vi "v5.1.vi"() -> ()   [LabVIEW 2018]
uses:
  <vilib>/DAQmx/read.llb/DAQmx Read (Analog 1D DBL NChan 1Samp).vi
  <extravilib>/ChannelInstances/High Speed Stream-c(a[.](c(dbl,dbl,dbl,dbl)),stamp,a[.](dbl),c(dbl,dbl,dbl,dbl,dbl,dbl,dbl))/_Read For Replicate.vi
  <extravilib>/ChannelInstances/High Speed Stream-c(a[.](c(dbl,dbl,dbl,dbl)),stamp,a[.](dbl),c(dbl,dbl,dbl,dbl,dbl,dbl,dbl))/Instantiate.vi
  <extravilib>/ChannelInstances/High Speed Stream-c(a[.](c(dbl,dbl,dbl,dbl)),stamp,a[.](dbl),c(dbl,dbl,dbl,dbl,dbl,dbl,dbl))/)Channel.vi
  <extravilib>/ChannelInstances/High Speed Stream-c(a[.](c(dbl,dbl,dbl,dbl)),stamp,a[.](dbl),c(dbl,dbl,dbl,dbl,dbl,dbl,dbl))/Abort Signal/Init Signal.vi
  <vilib>/Utility/file.llb/Write Delimited Spreadsheet (string).vi
  <vilib>/DAQmx/create/channels.llb/DAQmx Create Channel (AI-Temperature-Thermocouple).vi
  <vilib>/DAQmx/configure/timing.llb/DAQmx Timing (Sample Clock).vi
  <vilib>/DAQmx/miscellaneous.llb/DAQmx Fill In Error Info.vi
  <extravilib>/ChannelInstances/High Speed Stream-c(a[.](c(dbl,dbl,dbl,dbl)),stamp,a[.](dbl),c(dbl,dbl,dbl,dbl,dbl,dbl,dbl)).lvlib
  <resource>/objmgr/daqmx.rc
panel:
  in  "stop":bool
  in  "Species List":string[][](table)=[["Custom", "9999999999"], ["Methanol", "6.47"], ["Butanol", "11.2"], ["Diesel", "14.5"], ["Gasoline", "14.7"], ["Propane", "15.67"], ["Methane", "13.19"], ["Hydrogen", "34.3"], ["Ammonia", "6.0466"], ["Pentane", "15.32"], ["Butane", "14.98"], ["Hexane", "15.24"], ["Ethanol", "9"]]
  in  "Tab Control":enum32{"Live Data", "AFR Info", "Setup Lines"}(tab)
  out "Flowrate Data":T1(array[cluster])
  out "AFR Display":T2(array[cluster])
  in  "Line Setup":T3(array[cluster])
  out "Actual Sample Rate":dbl
  out "Export Timestamp":timestamp format="%<%H:%M:%S>T"
  out "Rig Temperatures":T4
  out "UI Timestamp":timestamp format="%<%X\n%x>T"
  out "DAQ Timestamp":timestamp format="%<%H:%M:%S>T"
  in  "file path (dialog if empty)":path
  out "Export Loop Status":T5(ring)
  in  "Start Recording?":bool
  in  "Stop Recording?":bool
  in  "Flowrate Control":dbl
  out "Aquisition Loop Status":T6(ring)
  in  "OK Button":bool
  in  "DAQ Properties":cluster{"Sample Rate [Hz]":dbl}={"Sample Rate [Hz]"=1.0} {"Sample Rate [Hz]" min=0.1 max=10000.0 step=0.1}
  # "Live \n Live Line Data"
  # "Air-to-Fuel Ratios for each Line"
  # "Line Setup"
  # "Rig Temperatures [ °C]"
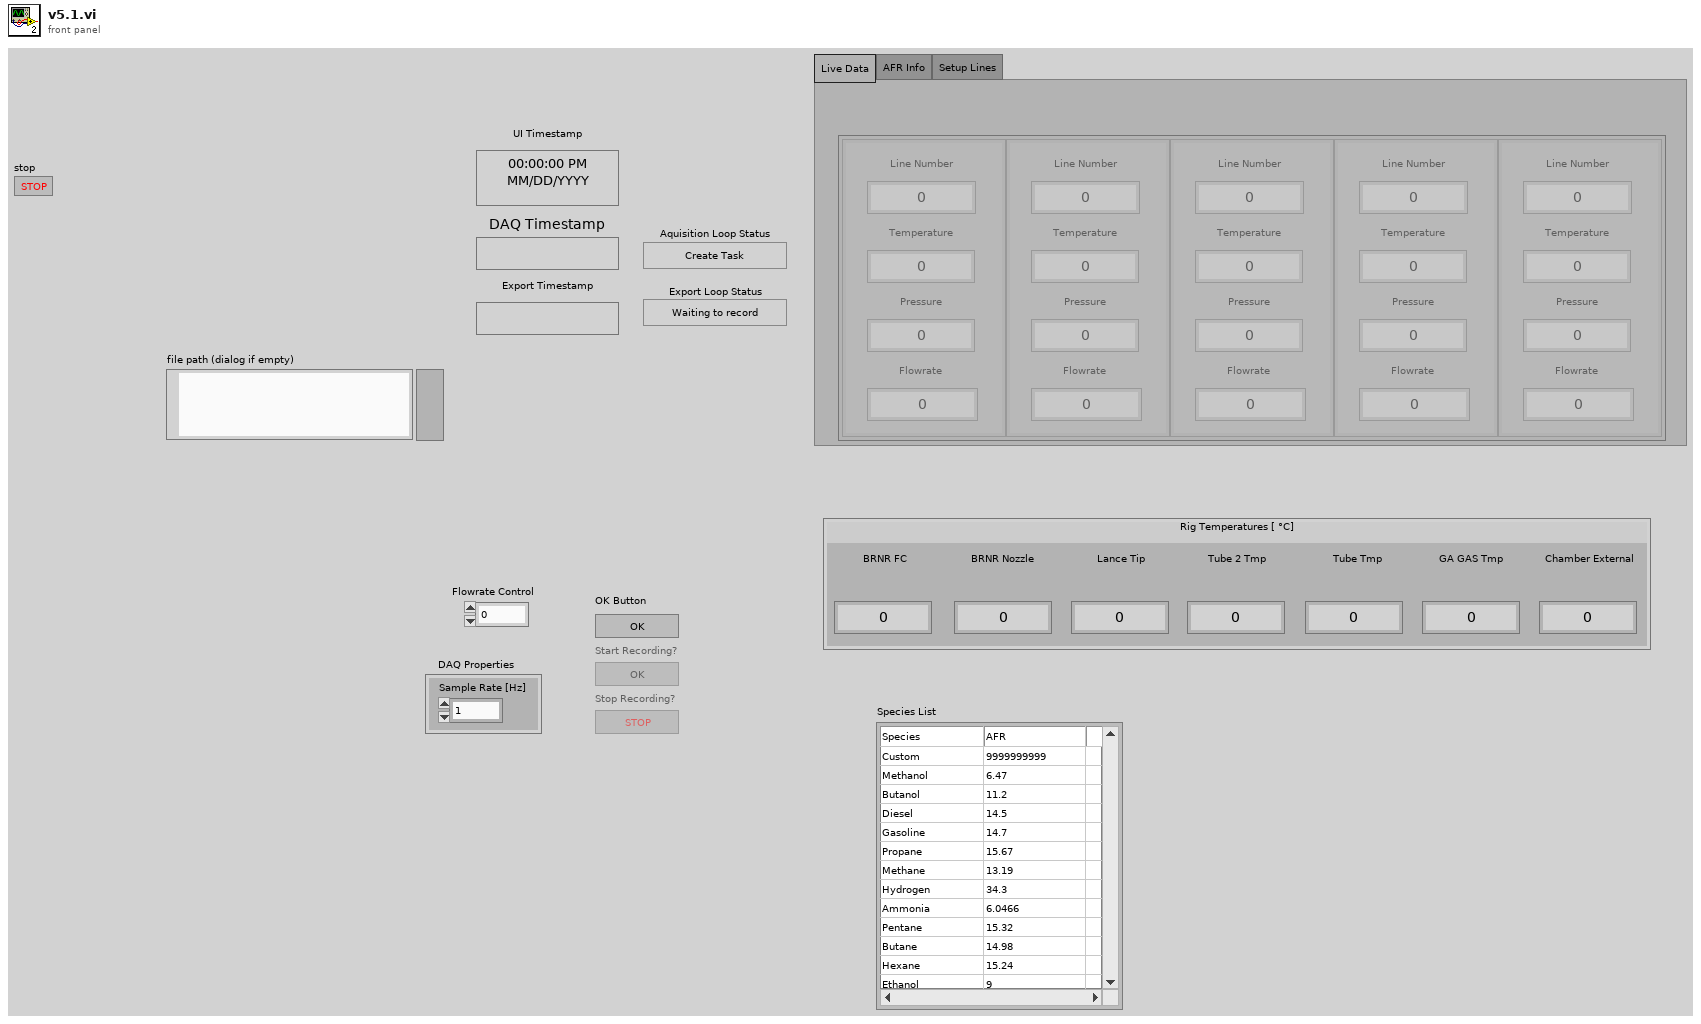
[diagram p1: front panel]
types:
  T1 = cluster{"Line Number":dbl, "Temperature":dbl, "Pressure":dbl, "Flowrate":dbl}[]
  T2 = cluster{"Line Number":i32, "AFR":dbl, "Species":enum16{"Methanol", "Ethanol", "Butanol", "Diesel", "Gasoline", "Propane", "Methane", "Hydrogen", "Pentane", "Butane", "Hexane", "Custom"}}[]
  T3 = cluster{"Custom AFR":dbl, "Species":enum16{"Methanol", "Ethanol", "Butanol", "Diesel", "Gasoline", "Propane", "Methane", "Hydrogen", "Pentane", "Butane", "Hexane", "Custom"}}[]
  T4 = cluster{"BRNR FC":dbl, "BRNR Nozzle":dbl, "Lance Tip":dbl, "Tube 2 Tmp":dbl, "Tube Tmp":dbl, "GA GAS Tmp":dbl, "Chamber External":dbl}
  T5 = enum16{"Waiting to record", "Creating Spreadsheet", "Recording", "Finished Recording"}
  T6 = enum16{"Create Task", "Change Settings", "Check Settings", "Read Data", "End Task"}
  T7 = enum8{"Enabled", "Disabled", "Disabled and Grayed Out"}
  T8 = cluster{"Line":i32, "AFR":dbl, "Species":enum16{"Methanol", "Ethanol", "Butanol", "Diesel", "Gasoline", "Propane", "Methane", "Hydrogen", "Pentane", "Butane", "Hexane", "Custom"}}
  T9 = enum16{"Methanol", "Ethanol", "Butanol", "Diesel", "Gasoline", "Propane", "Methane", "Hydrogen", "Pentane", "Butane", "Hexane", "Custom"}
  T10 = cluster{"Flowrate Data":cluster{"Line Number":dbl, "Temperature":dbl, "Pressure":dbl, "Flowrate":dbl}[], "Current Time":timestamp, "DAQmx Data":dbl[], "Rig Temperatures":cluster{"BRNR FC":dbl, "BRNR Nozzle":dbl, "Lance Tip":dbl, "Tube 2 Tmp":dbl, "Tube Tmp":dbl, "GA GAS Tmp":dbl, "Chamber External Temp":dbl}}
  T11 = cluster{"BRNR FC":dbl, "BRNR Nozzle":dbl, "Lance Tip":dbl, "Tube 2 Tmp":dbl, "Tube Tmp":dbl, "GA GAS Tmp":dbl, "Chamber External Temp":dbl}
  T12 = typedef "High Speed Stream-c(a[.](c(dbl,dbl,dbl,dbl)),stamp,a[.](dbl),c(dbl,dbl,dbl,dbl,dbl,dbl,dbl)).lvlib/)Channel.ctl" = refnum<queue>
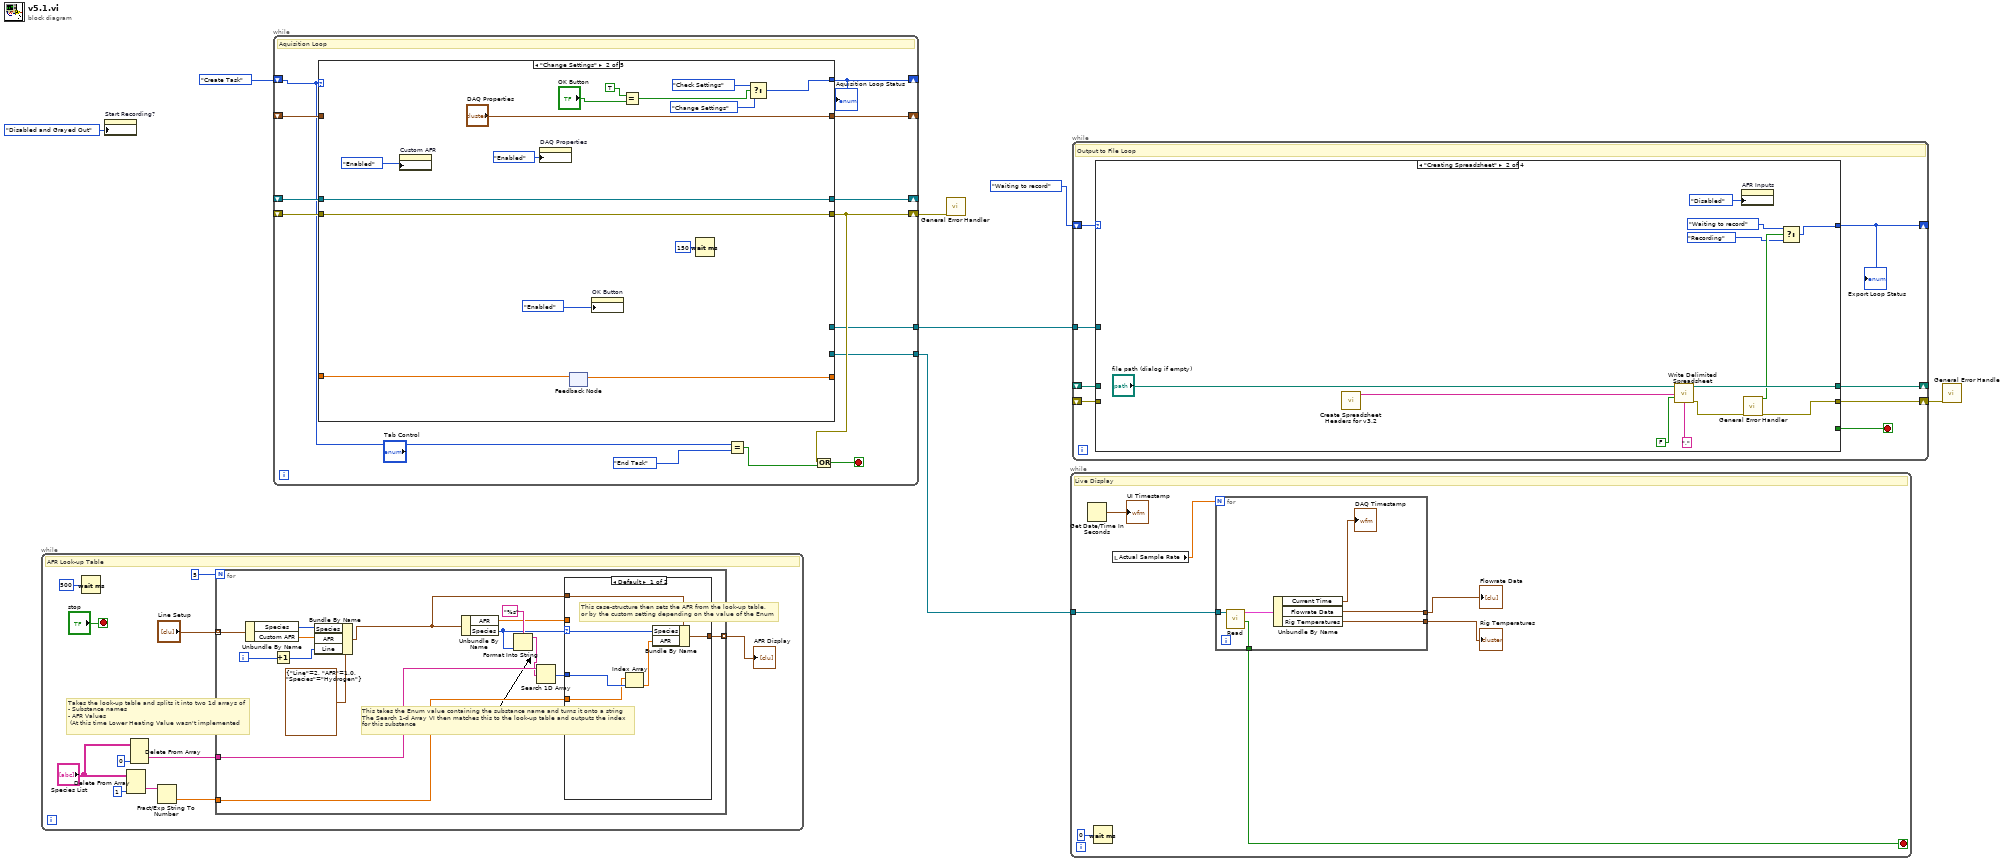
[diagram p0: block diagram]
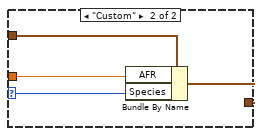
[diagram p2: hidden frame]
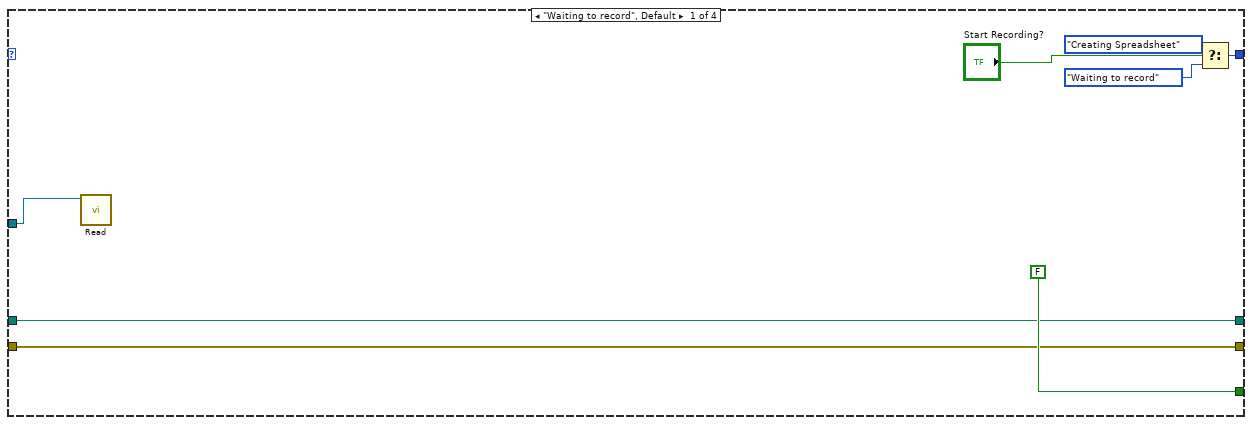
[diagram p3: hidden frame]
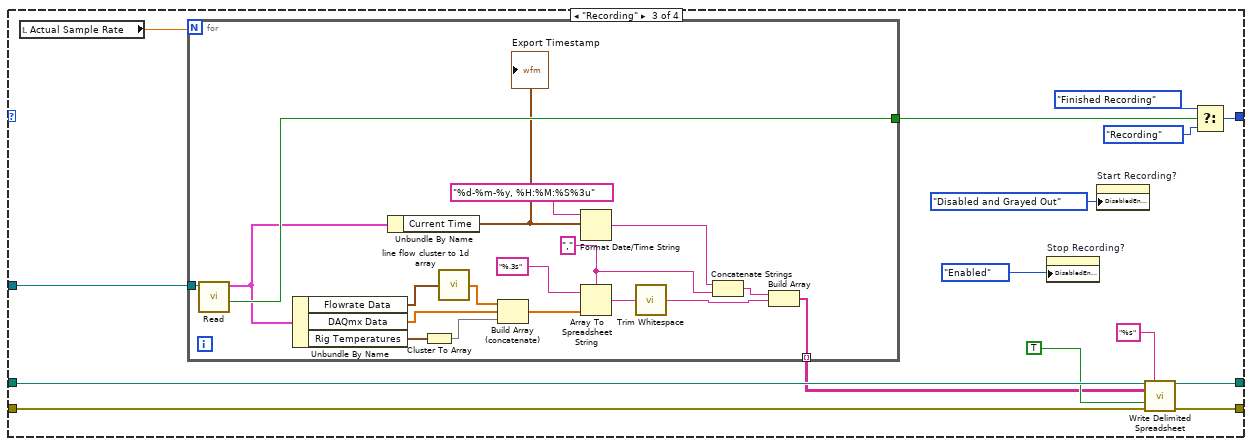
[diagram p4: hidden frame]
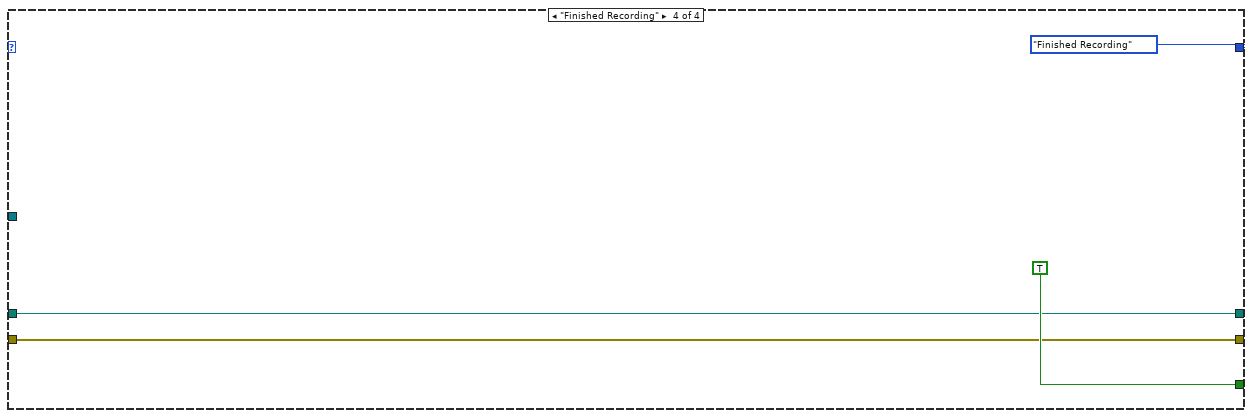
[diagram p5: hidden frame]
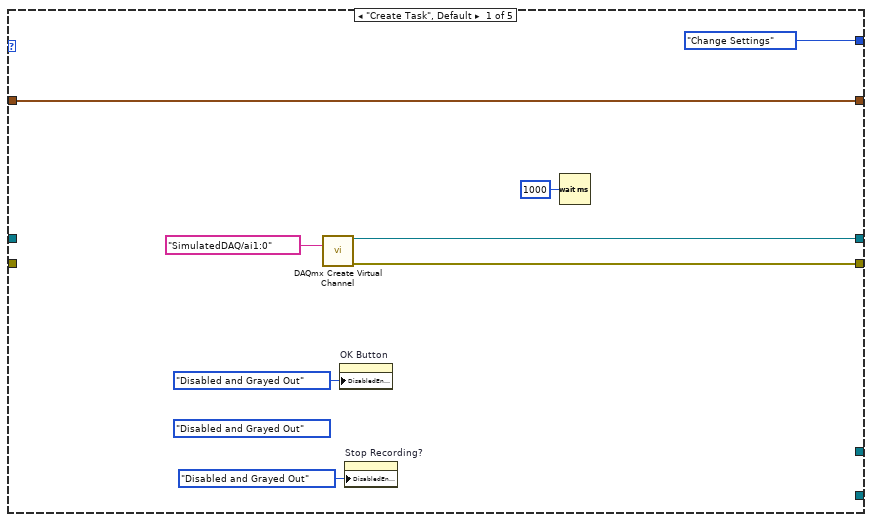
[diagram p6: hidden frame]
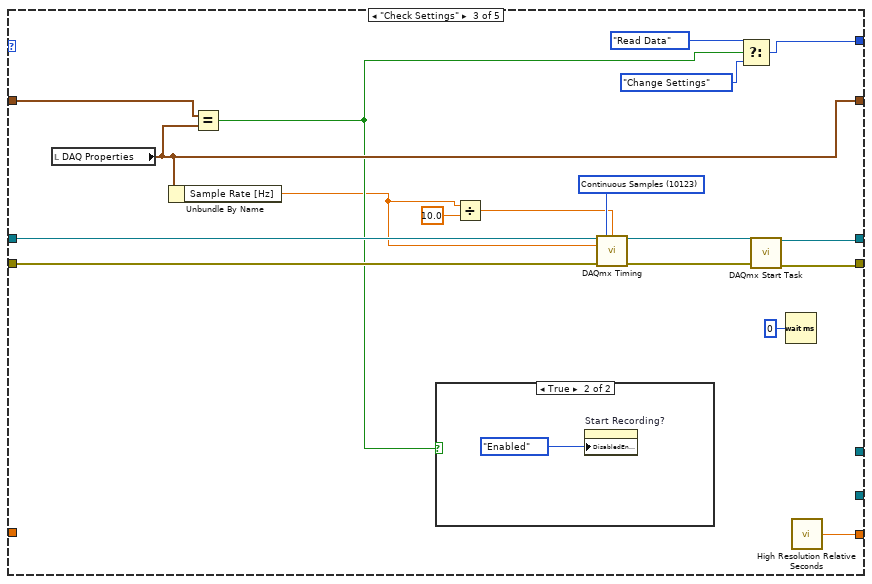
[diagram p7: hidden frame]
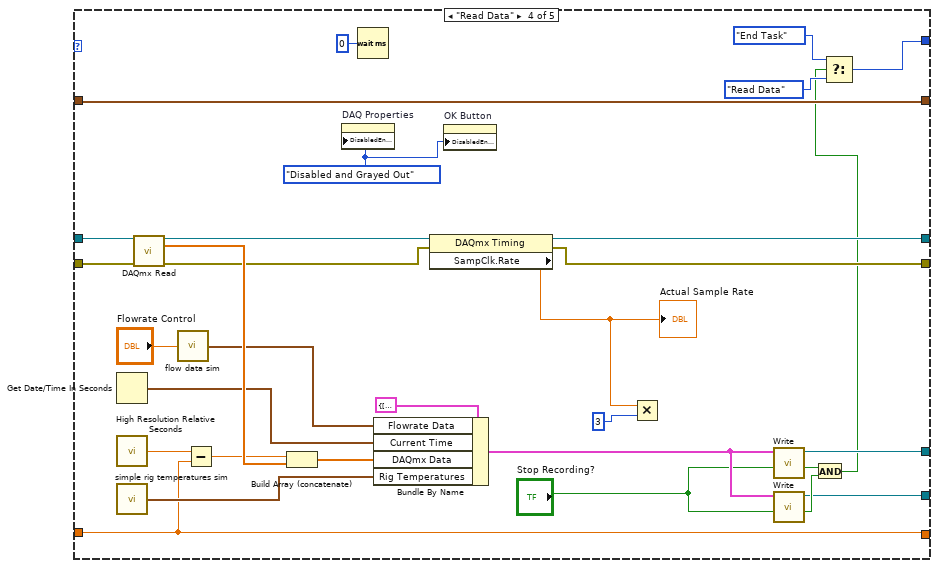
[diagram p9: hidden frame]
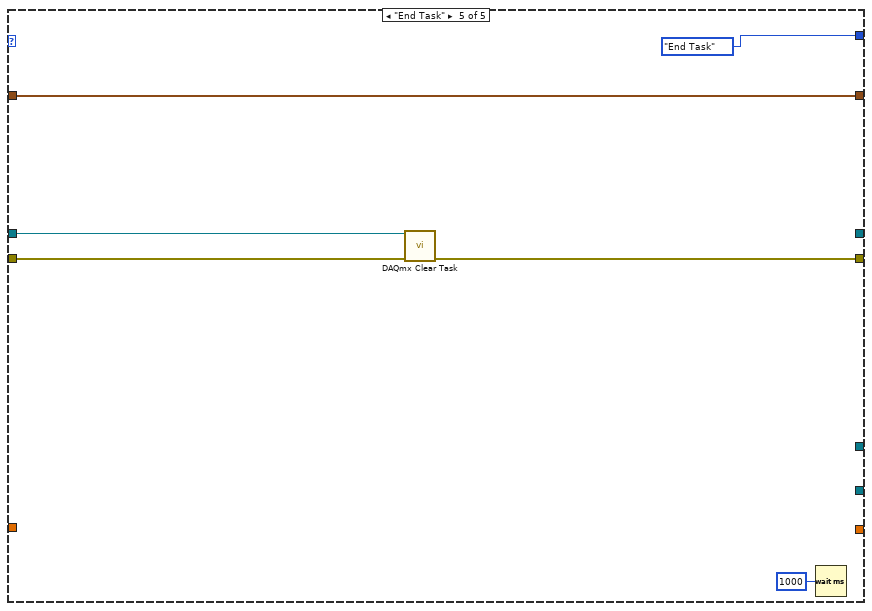
[diagram p10: hidden frame]
diagram:
  n1 = while {
    stop <- "stop" stop-if-true
    # "This case-structure then sets the AFR from the look-up table,\nor by the custom setting depending on the value of the Enum"
    # "Takes the look-up table and splits it into two 1d arrays of \n- Substance names \n- AFR Values\n (At this time Lower Heating Value wasn't implemented"
    # "AFR Look-up Table"
    n2 = Wait (ms)(milliseconds to wait=u32 500) -> ()  [unwired: 1 out]
    n3 = Delete From Array(array="Species List", index (col)=1 ("disabled index (col)")) -> (deleted portion=w13:string[])  [unwired: 2 in, 1 out]
    n4 = Delete From Array(array="Species List", index (col)=0) -> (deleted portion=w14:string[])  [unwired: 2 in, 1 out]
    n5 = Fract/Exp String To Number(string=w13) -> (number=w12:dbl[])  [unwired: 3 in, 1 out]
    n6 = for {
      N: 5 -> [_]
      tunnel: w14 -> [w32]
      tunnel: w12 -> [w29]
      tunnel: [w27] -> w10 mode=indexing
      tunnel: "Line Setup" -> [w21] mode=indexing
      i -> [w20]
      # "This takes the Enum value containing the substance name and turns it onto a string\nThe Search 1-d Array VI then matches this to the look-up table and outputs the index \nfor this substance"
      n7 = Unbundle By Name(w21) -> ("Species"=w25:T9, "Custom AFR"=w24:dbl)
      n8 = Increment(x=w20) -> (x+1=w22:i32)
      n9 = Bundle By Name(cluster=T8 {"Line"=2, "AFR"=1.0, "Species"=enum."Hydrogen"} ("AFR Inputs"), "Species"=w25, "AFR"=w24, "Line"=w22) -> (w19:T8)
      n10 = Unbundle By Name(w19) -> ("AFR"=w30:dbl, "Species"=w26:T9)
      n11 = Format Into String(format string="%s", w26) -> (resulting string=w31:string)  [unwired: 2 in, 1 out]
      n12 = Search 1D Array(1D array=w32, element=w31) -> (index of element=w28:i32)  [unwired: 1 in]
      n13 = case shown="Default" w26 {
        selector: w26 -> [w39 w42]
        tunnel: w30 -> [_ w43]
        tunnel: w29 -> [w37 _]
        tunnel: w28 -> [w38 _]
        tunnel: [w35 w41] -> w27
        tunnel: w19 -> [w34 w40]
        frame Default {
          n14 = Index Array(array=w37, index=w38) -> (element=w36:dbl)
          n15 = Bundle By Name(cluster=w34, "Species"=w39, "AFR"=w36) -> (w35:T8)
        }
        frame "Custom" {
          n16 = Bundle By Name(cluster=w40, "AFR"=w43, "Species"=w42) -> (w41:T8)
        }
      }
    }
    "AFR Display" <- w10
  }
  n17 = property on="Start Recording?" class="Bool"("DisabledEnum"=T7."Disabled and Grayed Out" ("Disabled")) -> ()  [unwired: 2 in, 2 out]
  n18 = while {
    shift-right: [w53] -> _
    shift-left: T6."Create Task" -> [w49]
    shift-right: [w58] -> _
    shift-left: _ -> [w56]
    shift-right: [w52] -> w3
    shift-left: _ -> [w55]
    shift-right: [w57] -> _
    shift-left: _ -> [w54]
    tunnel: [w48] -> w5
    tunnel: [w47] -> w1
    stop <- w44 stop-if-true
    # "Aquisition Loop"
    n19 = feedback #1() -> (w45:dbl)  [unwired: 1 in]
    n20 = case shown="\"Change Settings\"" w49 {
      tunnel: [w66 w79 w87 w109 _] -> w58
      tunnel: [w65 w78 w86 w110 w135] -> w52
      tunnel: [T6."Change Settings" w72 w93 w125 T6."End Task"] -> w53
      tunnel: [w62 "DAQ Properties" w90 w127 w134] -> w57
      tunnel: w56 -> [_ w79 w92 w129 w132]
      tunnel: w55 -> [_ w78 w91 w128 w131]
      tunnel: w54 -> [w62 _ w97 w127 w134]
      tunnel: [_ _ _ w116 _] -> w48
      tunnel: [_ _ _ w107 _] -> w47
      tunnel: [_ _ w80 w102 _] -> w46
      tunnel: w45 -> [_ _ _ w102 _]
      frame "Create Task", Default {
        (unwired) T7."Disabled and Grayed Out" ("Disabled")
        n21 = call-poly <vilib>:"DAQmx Create Virtual Channel.vi"("physical channels"=tag "SimulatedDAQ/ai1:0") -> ("task out"=w66:refnum<k21>, "error out"=w65:errorcluster)  [unwired: 13 in]
        n22 = property on="OK Button" class="Bool"("DisabledEnum"=T7."Disabled and Grayed Out" ("Disabled")) -> ()  [unwired: 2 in, 2 out]
        n23 = property on="Stop Recording?" class="Bool"("DisabledEnum"=T7."Disabled and Grayed Out" ("Disabled")) -> ()  [unwired: 2 in, 2 out]
        n24 = Wait (ms)(milliseconds to wait=u32 1000) -> ()  [unwired: 1 out]
      }
      frame "Change Settings" {
        n25 = property on="Custom AFR" class="DigNum (strict)"("DisabledEnum"=T7."Enabled" ("Disabled")) -> ()  [unwired: 2 in, 2 out]
        n26 = property on="DAQ Properties" class="Clust (strict)"("DisabledEnum"=T7."Enabled" ("Disabled")) -> ()  [unwired: 2 in, 2 out]
        n27 = property on="OK Button" class="Bool"("DisabledEnum"=T7."Enabled" ("Disabled")) -> ()  [unwired: 2 in, 2 out]
        n28 = Equal?(x=TRUE, y="OK Button") -> (x = y?=w74:bool)
        n29 = Wait (ms)(milliseconds to wait=u32 150) -> ()  [unwired: 1 out]
        n30 = Select(t=T6."Check Settings", s=w74, f=T6."Change Settings") -> (s? t:f=w72:T6)
      }
      frame "Check Settings" {
        w85 = 10123 items=["Finite Samples"=10178, "Continuous Samples"=10123, "Hardware Timed Single Point"=12522] ("sample mode")
        n31 = local read "DAQ Properties"() -> (w90:cluster{"Sample Rate [Hz]":dbl})
        n32 = Unbundle By Name(w90) -> ("Sample Rate [Hz]"=w82:dbl)
        n33 = Equal?(x=w97, y=w90) -> (x = y?=w84:bool)
        n34 = case shown="True" w84 {
          frame False {
          }
          frame True {
            n35 = property on="Start Recording?" class="Bool"("DisabledEnum"=T7."Enabled" ("Disabled")) -> ()  [unwired: 2 in, 2 out]
          }
        }
        n36 = Divide(x=w82, y=10.0) -> (x/y=w81:dbl)
        n37 = call-poly <vilib>:"DAQmx Timing.vi"("task/channels in"=w92, "sample mode"=w85, "samples per channel"=w81, "rate"=w82, "error in"=w91) -> ("task out"=w89:refnum<k21>, "error out"=w88:errorcluster)  [unwired: 9 in]
        n38 = Select(t=T6."Read Data", s=w84, f=T6."Change Settings") -> (s? t:f=w93:T6)
        n39 = call <vilib>:"DAQmx Start Task.vi"("task/channels in"=w89, "error in"=w88) -> ("task out"=w87:refnum<k21>, "error out"=w86:errorcluster)  [unwired: 12 in]
        n40 = Wait (ms)(milliseconds to wait=u32 0) -> ()  [unwired: 1 out]
        n41 = call <vilib>:"High Resolution Relative Seconds.vi"() -> ("relative seconds"=w80:dbl)
      }
      frame "Read Data" {
        w115 = T7."Disabled and Grayed Out" ("Disabled")
        n42 = Get Date/Time In Seconds() -> (seconds since 1Jan1904=w119:timestamp)
        n43 = call <vilib>:"High Resolution Relative Seconds.vi"() -> ("relative seconds"=w106:dbl)
        n44 = call "simple rig temperatures sim.vi"() -> ("Rig Temperatures"=w117:T11)
        n45 = call-poly <vilib>:"DAQmx Read.vi"("task/channels in"=w129, "error in"=w128) -> ("task out"=w111:refnum<k21>, "data"=w122:dbl[], "error out"=w108:errorcluster)  [unwired: 11 in]
        n46 = call "flow data sim.vi"("Boondoggle Input"="Flowrate Control") -> ("Flowrate Data"=w118:T1)
        n47 = Subtract(x=w106, y=w102) -> (x-y=w103:dbl)
        n48 = Build Array (concatenate)(w103, w122) -> (w104:dbl[])
        n49 = property on="DAQ Properties" class="Clust (strict)"("DisabledEnum"=w115) -> ()  [unwired: 2 in, 2 out]
        n50 = Wait (ms)(milliseconds to wait=u32 0) -> ()  [unwired: 1 out]
        n51 = Bundle By Name(cluster=T10 {"Flowrate Data"=[{"Line Number"=1.0, "Temperature"=17.480721541683437, "Pressure"=24.0, "Flowrate"=0.0}, {"Line Number"=2.0, "Temperature"=21.850901927104296, "Pressure"=30.0, "Flowrate"=0.0}, {"Line Number"=3.0, "Temperature"=26.221082312525155, "Pressure"=36.0, "Flowrate"=0.0}, {"Line Number"=4.0, "Temperature"=30.591262697946018, "Pressure"=42.00000000000001, "Flowrate"=0.0}, {"Line Number"=5.0, "Temperature"=34.96144308336687, "Pressure"=48.0, "Flowrate"=0.0}], "Current Time"=timestamp(0 s since 1904-01-01), "DAQmx Data"=[], "Rig Temperatures"={"BRNR FC"=0.0, "BRNR Nozzle"=0.0, "Lance Tip"=0.0, "Tube 2 Tmp"=0.0, "Tube Tmp"=0.0, "GA GAS Tmp"=0.0, "Chamber External Temp"=0.0}}, "Flowrate Data"=w118, "Current Time"=w119, "DAQmx Data"=w104, "Rig Temperatures"=w117) -> (w114:T10)
        n52 = property class="DAQmx Timing"(reference=w111, error in=w108) -> (reference out=w109:refnum<k21>, error out=w110:errorcluster, "SampClk.Rate"=w101:dbl)
        "Actual Sample Rate" <- w101
        n53 = property on="OK Button" class="Bool"("DisabledEnum"=w115) -> ()  [unwired: 2 in, 2 out]
        n54 = Multiply(x=w101, y=3) -> ()  [unwired: 1 out]
        n55 = call <extravilib>:"Write.vi"("last element? (F)"="Stop Recording?", "element"=w114) -> ("done?"=w113:bool, "channel"=w116:T12)  [unwired: 7 in, 1 out]
        n56 = call <extravilib>:"Write.vi"("last element? (F)"="Stop Recording?", "element"=w114) -> ("done?"=w112:bool, "channel"=w107:T12)  [unwired: 7 in, 1 out]
        n57 = And(x=w113, y=w112) -> (x .and. y?=w105:bool)
        n58 = Select(t=T6."End Task", s=w105, f=T6."Read Data") -> (s? t:f=w125:T6)
      }
      frame "End Task" {
        n59 = call <vilib>:"DAQmx Clear Task.vi"("task in"=w132, "error in"=w131) -> ("error out"=w135:errorcluster)  [unwired: 13 in]
        n60 = Wait (ms)(milliseconds to wait=u32 1000) -> ()  [unwired: 1 out]
      }
    }
    "Aquisition Loop Status" <- w53
    n61 = feedback-in #1(w46) -> ()
    n62 = Equal?(x=w49, y=T6."End Task") -> (x = y?=w50:bool)
    n63 = Or(x=w52, y=w50) -> (x .or. y?=w44:bool)
  }
  n64 = call <vilib>:"General Error Handler.vi"("error in (no error)"=w3) -> ()  [unwired: 10 in, 5 out]
  n65 = while {
    tunnel: w1 -> [w139]
    stop <- w142 stop-if-true
    # "Live Display"
    n66 = Get Date/Time In Seconds() -> (seconds since 1Jan1904=→"UI Timestamp":timestamp)
    n67 = Wait (ms)(milliseconds to wait=u32 0) -> ()  [unwired: 1 out]
    n68 = local read "Actual Sample Rate"() -> (w138:dbl)
    n69 = for {
      N: w138 -> [_]
      tunnel: [w148] -> w142
      tunnel: w139 -> [w145]
      tunnel: [w144] -> w136
      tunnel: [w143] -> w137
      n70 = call <extravilib>:"Read.vi"("channel"=w145) -> ("done?"=w148:bool, "element"=w147:T10)  [unwired: 6 in, 3 out]
      n71 = Unbundle By Name(w147) -> ("Current Time"=→"DAQ Timestamp":timestamp, "Flowrate Data"=w144:T1, "Rig Temperatures"=w143:T11)
    }
    "Flowrate Data" <- w136
    "Rig Temperatures" <- w137
  }
  n72 = while {
    shift-right: [w156] -> _
    shift-left: T5."Waiting to record" -> [w155]
    tunnel: w5 -> [w153]
    shift-right: [w151] -> _
    shift-left: _ -> [w152]
    shift-right: [w150] -> w4
    shift-left: _ -> [w149]
    stop <- w154 stop-if-true
    # "Output to File Loop"
    n73 = case shown="\"Creating Spreadsheet\"" w155 {
      tunnel: [w161 w168 w190 T5."Finished Recording"] -> w156
      tunnel: [FALSE _ _ TRUE] -> w154
      tunnel: w153 -> [w157 _ w187 _]
      tunnel: w152 -> [w159 _ w184 w211]
      tunnel: [w159 w176 w185 w211] -> w151
      tunnel: [w158 w170 w180 w210] -> w150
      tunnel: w149 -> [w158 _ w183 w210]
      frame "Waiting to record", Default {
        n74 = call <extravilib>:"Read.vi"("channel"=w157) -> ()  [unwired: 6 in, 5 out]
        n75 = Select(t=T5."Creating Spreadsheet", s="Start Recording?", f=T5."Waiting to record") -> (s? t:f=w161:T5)
      }
      frame "Creating Spreadsheet" {
        n76 = call "Create Spreadsheet Headers for v3.2.vi"() -> ("Array"=w175:string[])  [unwired: 11 in]
        n77 = call-poly <vilib>:"Write Delimited Spreadsheet.vi"("file path (dialog if empty)"="file path (dialog if empty)", "1D data"=w175, "append to file? (new file:F)"=FALSE, "delimiter (\\t)"="," ("delimiter (\\t)")) -> ("new file path (Not A Path if cancelled)"=w176:path, "error out"=w171:errorcluster)  [unwired: 10 in]
        n78 = property on="AFR Inputs" class="Clust (strict)"("DisabledEnum"=T7."Disabled" ("Disabled")) -> ()  [unwired: 2 in, 2 out]
        n79 = call <vilib>:"General Error Handler.vi"("error in (no error)"=w171) -> ("error?"=w169:bool, "error out"=w170:errorcluster)  [unwired: 10 in, 3 out]
        n80 = Select(t=T5."Waiting to record", s=w169, f=T5."Recording") -> (s? t:f=w168:T5)
      }
      frame "Recording" {
        n81 = local read "Actual Sample Rate"() -> (w177:dbl)
        n82 = for {
          N: w177 -> [_]
          tunnel: w187 -> [w208]
          tunnel: [w207] -> w186
          tunnel: [w192] -> w178 mode=indexing
          w197 = "," ("delimiter (Tab)")
          n83 = call <extravilib>:"Read.vi"("channel"=w208) -> ("done?"=w207:bool, "element"=w205:T10)  [unwired: 6 in, 3 out]
          n84 = Unbundle By Name(w205) -> ("Flowrate Data"=w206:T1, "DAQmx Data"=w203:dbl[], "Rig Temperatures"=w209:T11)
          n85 = Unbundle By Name(w205) -> ("Current Time"=w198:timestamp)
          "Export Timestamp" <- w198
          n86 = Cluster To Array(cluster=w209) -> (array=w204:dbl[])
          n87 = call "line flow cluster to 1d array.vi"("Flowrate Data"=w206) -> ("Array"=w202:dbl[])
          n88 = Build Array (concatenate)(w202, w203, w204) -> (w195:dbl[])
          n89 = Format Date/Time String(time format string (%c)="%d-%m-%y, %H:%M:%S%3u", seconds (now)=w198) -> (date/time string=w196:string)  [unwired: 1 in]
          n90 = Array To Spreadsheet String(delimiter (Tab)=w197, array=w195, 3:"%.3s" ("format string")) -> (spreadsheet string=w201:string)
          n91 = call <vilib>:"Trim Whitespace.vi"("string"=w201) -> ("trimmed string"=w193:string)  [unwired: 1 in]
          n92 = Concatenate Strings(w196, w197) -> (w194:string)
          n93 = Build Array(w194, w193) -> (w192:string[])
        }
        n94 = property on="Stop Recording?" class="Bool"("DisabledEnum"=T7."Enabled" ("Disabled")) -> ()  [unwired: 2 in, 2 out]
        n95 = property on="Start Recording?" class="Bool"("DisabledEnum"=T7."Disabled and Grayed Out" ("Disabled")) -> ()  [unwired: 2 in, 2 out]
        n96 = call-poly <vilib>:"Write Delimited Spreadsheet.vi"("file path (dialog if empty)"=w184, "format (%s)"="%s", "2D data"=w178, "append to file? (new file:F)"=TRUE, "error in (no error)"=w183) -> ("new file path (Not A Path if cancelled)"=w185:path, "error out"=w180:errorcluster)  [unwired: 9 in]
        n97 = Select(t=T5."Finished Recording", s=w186, f=T5."Recording") -> (s? t:f=w190:T5)
      }
      frame "Finished Recording" {
      }
    }
    "Export Loop Status" <- w156
  }
  n98 = call <vilib>:"General Error Handler.vi"("error in (no error)"=w4) -> ()  [unwired: 10 in, 5 out]
